vi "Untitled 12.vi"() -> ()   [LabVIEW 2021]
uses:
  src/Expression.ctl
  src/ExpressionType.ctl
panel:
  out "Expression out":T1
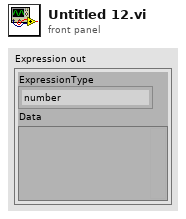
[diagram p1: front panel]
types:
  T1 = typedef "Expression.ctl" = cluster{"ExpressionType":T2, "Data":variant}
  T2 = typedef "ExpressionType.ctl" = enum16{"number", "string", "symbol", "primitive", "list", "closure", "nil", "error"}
  T3 = cluster{"Parent Environment":variant, "map":map{string, T1}}
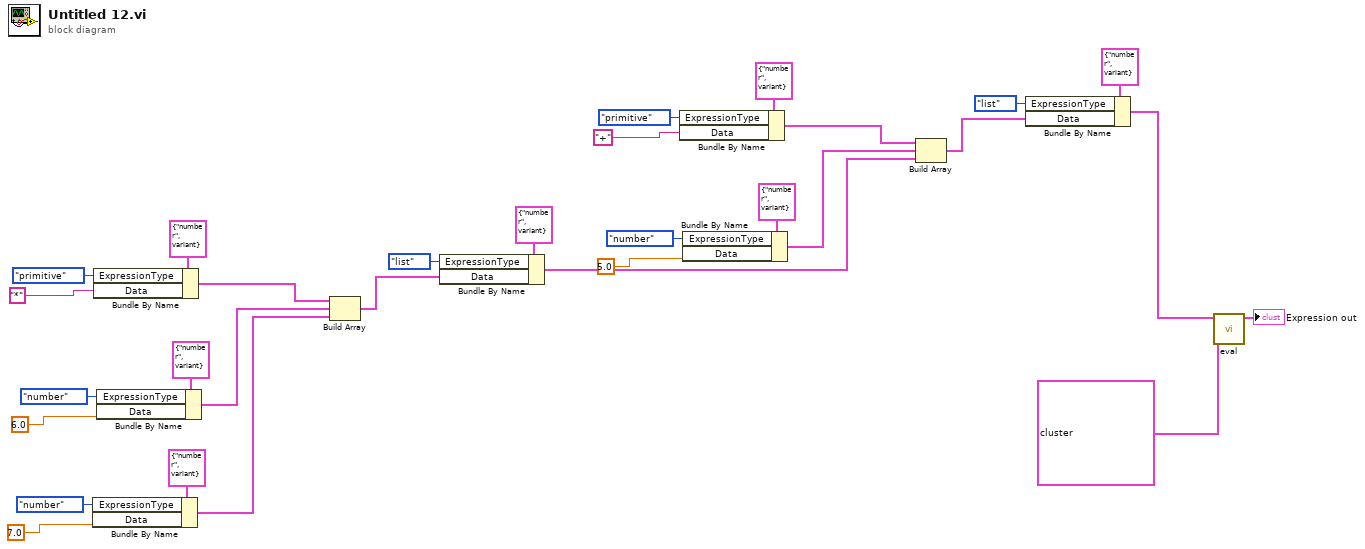
[diagram p0: block diagram]
diagram:
  n1 = Bundle By Name(cluster=T1 {"ExpressionType"=enum."number", "Data"=variant} ("Expression in"), "ExpressionType"=ExpressionType."number", "Data"=7.0) -> (w16:T1)
  n2 = Bundle By Name(cluster=T1 {"ExpressionType"=enum."number", "Data"=variant} ("Expression in"), "ExpressionType"=ExpressionType."primitive", "Data"="*") -> (w18:T1)
  n3 = Bundle By Name(cluster=T1 {"ExpressionType"=enum."number", "Data"=variant} ("Expression in"), "ExpressionType"=ExpressionType."number", "Data"=6.0) -> (w17:T1)
  n4 = Build Array(w18, w17, w16) -> (w28:T1[])
  n5 = Bundle By Name(cluster=T1 {"ExpressionType"=enum."number", "Data"=variant} ("Expression in"), "ExpressionType"=ExpressionType."list", "Data"=w28) -> (w2:T1)
  n6 = Bundle By Name(cluster=T1 {"ExpressionType"=enum."number", "Data"=variant} ("Expression in"), "ExpressionType"=ExpressionType."primitive", "Data"="+") -> (w4:T1)
  n7 = Bundle By Name(cluster=T1 {"ExpressionType"=enum."number", "Data"=variant} ("Expression in"), "ExpressionType"=ExpressionType."number", "Data"=5.0) -> (w3:T1)
  n8 = Build Array(w4, w3, w2) -> (w11:T1[])
  n9 = Bundle By Name(cluster=T1 {"ExpressionType"=enum."number", "Data"=variant} ("Expression in"), "ExpressionType"=ExpressionType."list", "Data"=w11) -> (w1:T1)
  n10 = call "eval.vi"("Environment"=T3 {"Parent Environment"=variant, "map"={}}, "Expression in"=w1) -> ("Expression out"=→"Expression out":T1)  [unwired: 7 in]
